vi "Measurement Logic.vi"() -> ()   [LabVIEW 2021, in "Single Tone_Audio DAC.lvlib"]
uses:
  Single Tone_Audio DAC.lvlib
  <vilib>/PDM Acquisition Toolkit/host/Classes/Channels/I2S Ouput/Controls/GenerationChannelProperties.ctl
  <vilib>/PDM Acquisition Toolkit/host/Classes/Channels/I2S Ouput/I2S Output Channel.lvclass
  <vilib>/PDM Acquisition Toolkit/host/Classes/Tasks/I2S Output/Control/SignalProperties.ctl
  <vilib>/PDM Acquisition Toolkit/host/Classes/Tasks/I2S Output/I2S Output Task.lvclass
  shared/controls/Digital Initialize Settings.ctl
  shared/controls/Analog Initialize Settings.ctl
  shared/controls/Single Tone Measurement Settings.ctl
  shared/controls/Single Tone Units.ctl
  Measurement Results.ctl
  shared/controls/Single Tone Filter Settings.ctl
  Measurement Configuration.ctl
  <vilib>/MeasurementLink/MeasurementLink Measurement Server/Measure Call Context/Measure Call Context.lvclass
panel:
  out "measure call context out":refnum<class "Measure Call Context.lvclass">
  in  "measure call context in":refnum<class "Measure Call Context.lvclass">
  out "measurement results":T1 {"Gain" format="%_6g"; "THD" format="%_6g"; "THD+N" format="%_6g"; "SNR" format="%_6g"; "SFDR (dBc)" format="%_6g"; "Dynamic range (dB)" format="%_6g"; "Phase (deg)" format="%_6g"; "Amplitude (dB)" format="%_6g"; "Amplitude (V)" format="%_6g"; "Frequency (Hz)" format="%_6g"; "df" format="%_6g"; "f0" format="%_6g"; "dt" format="%_6g"; "Frequency domain" format="%_6g"; "Time domain" format="%_6g"}
  in  "measurement configuration":T2={"Frequency (Hz)"=1000.0, "Protocol file"="C:\\Users\\Public\\Documents\\National Instruments\\AudioDAC\\ProtocolConfig\\I2SDEfault.dsgcfg", "Digital audio channel"="7821/PCMo 16", "Master clock channel"="7821/PCMo 24", "Output level"=0.0, "Output level units"="dBFS", "Output range (Vpk-pk)"=5.74, "Acquisition channel"="4468/ai0", "Sample rate (Hz)"=51200.0, "Min measurement cycles"=0, "Min measurement time (s)"=1.0, "Min settling cycles"=0, "Min settling time (s)"=0.5, "Highpass filter"="AC", "Lowpass filter"="AES17_20kHz", "Weighting filter"="A-weighting", "Band start (Hz)"=20.0, "Band stop (Hz)"=20000.0, "SNR units"="dB", "THD+N units"="dB", "THD units"="dB", "Gain units"="dB"} {"Band stop (Hz)" format="%#_6pHz"; "Band start (Hz)" format="%#_6pHz"; "Min settling time (s)" format="%#_6ps"; "Min measurement time (s)" format="%#_6ps"; "Sample rate (Hz)" format="%#_6pHz"; "Output range (Vpk-pk)" format="%.3p Vpk-pk"; "Output level" format="%#_6p"; "Frequency (Hz)" format="%#_6pHz"}
  out "error out":errorcluster
  in  "error in":errorcluster
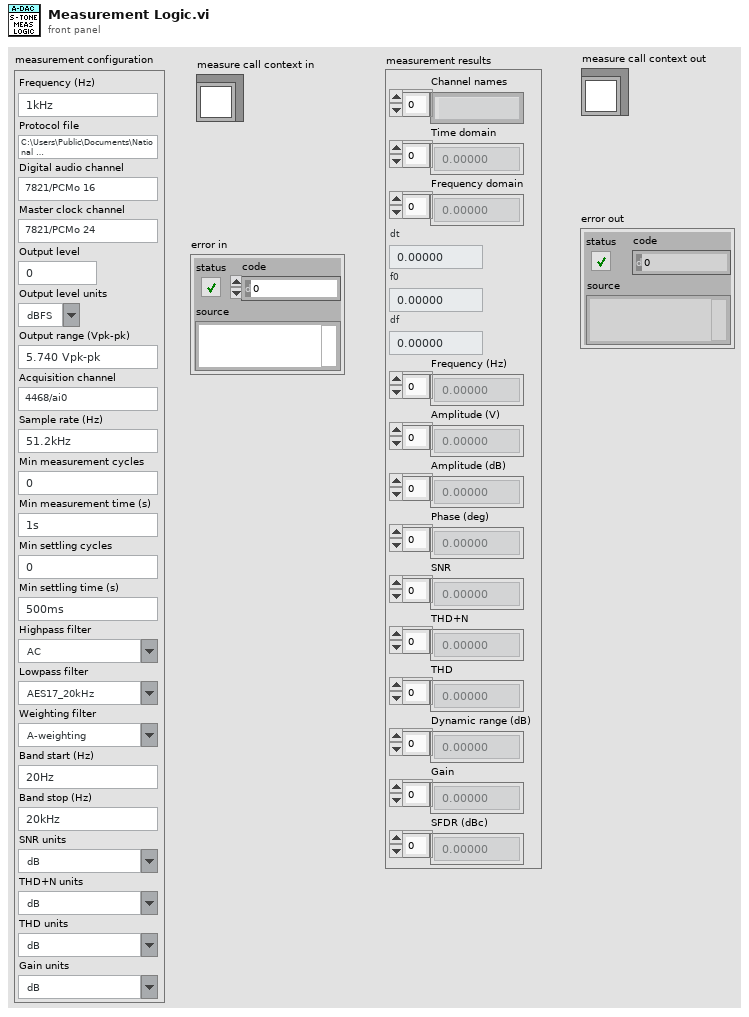
[diagram p1: front panel]
types:
  T1 = typedef "Single Tone_Audio DAC.lvlib/Measurement Results.ctl" = cluster{"Channel names":string[], "Time domain":dbl[], "Frequency domain":dbl[], "dt":dbl, "f0":dbl, "df":dbl, "Frequency (Hz)":dbl[], "Amplitude (V)":dbl[], "Amplitude (dB)":dbl[], "Phase (deg)":dbl[], "SNR":dbl[], "THD+N":dbl[], "THD":dbl[], "Dynamic range (dB)":dbl[], "Gain":dbl[], "SFDR (dBc)":dbl[]}
  T2 = typedef "Single Tone_Audio DAC.lvlib/Measurement Configuration.ctl" = cluster{"Frequency (Hz)":dbl, "Protocol file":string, "Digital audio channel":string, "Master clock channel":string, "Output level":dbl, "Output level units":string, "Output range (Vpk-pk)":dbl, "Acquisition channel":string, "Sample rate (Hz)":dbl, "Min measurement cycles":u32, "Min measurement time (s)":dbl, "Min settling cycles":u32, "Min settling time (s)":dbl, "Highpass filter":string, "Lowpass filter":string, "Weighting filter":string, "Band start (Hz)":dbl, "Band stop (Hz)":dbl, "SNR units":string, "THD+N units":string, "THD units":string, "Gain units":string}
  T3 = typedef "Single Tone Filter Settings.ctl" = cluster{"Highpass filter":string, "Lowpass filter":string, "Weighting filter":string}
  T4 = typedef "Single Tone Units.ctl" = cluster{"SNR units":string, "THD+N units":string, "THD units":string, "Gain units":string}
  T5 = typedef "Single Tone Measurement Settings.ctl" = cluster{"Band start":dbl, "Band stop":dbl, "Amplitude":dbl, "Frequency":dbl, "Full scale range":dbl}
  T6 = typedef "Analog Initialize Settings.ctl" = cluster{"analog acquisition channel":string, "samples per channel":i32, "sample rate":dbl}
  T7 = typedef "Digital Initialize Settings.ctl" = cluster{"digital channel list":string, "master clock channel list":string, "protocol settings file path":path, "signal parameters":T8}
  T8 = typedef "PDM Acquisition Class Library.lvlib/I2S Output Task.lvclass/SignalProperties.ctl" = cluster{"cyclic signal":dbl[], "channel parameters":T9[]}
  T9 = typedef "PDM Acquisition Class Library.lvlib/I2S Output Channel.lvclass/GenerationChannelProperties.ctl" = cluster{"cyclic period":dbl, "cyclic phase offset":dbl, "gain":dbl}
  T10 = typedef "PDM Acquisition Class Library.lvlib/PCM Output Task.lvclass/PCM Output Task DVR.ctl" = refnum<data-value>
  T11 = cluster{"channel":string, "frequency (Hz)":dbl, "amplitude (Vrms)":dbl, "amplitude (dBFS)":dbl, "phase (deg)":dbl, "SNR":dbl, "THD+N":dbl, "THD":dbl, "dynamic range (dB)":dbl, "gain":dbl, "SFDR (dBc)":dbl}[]
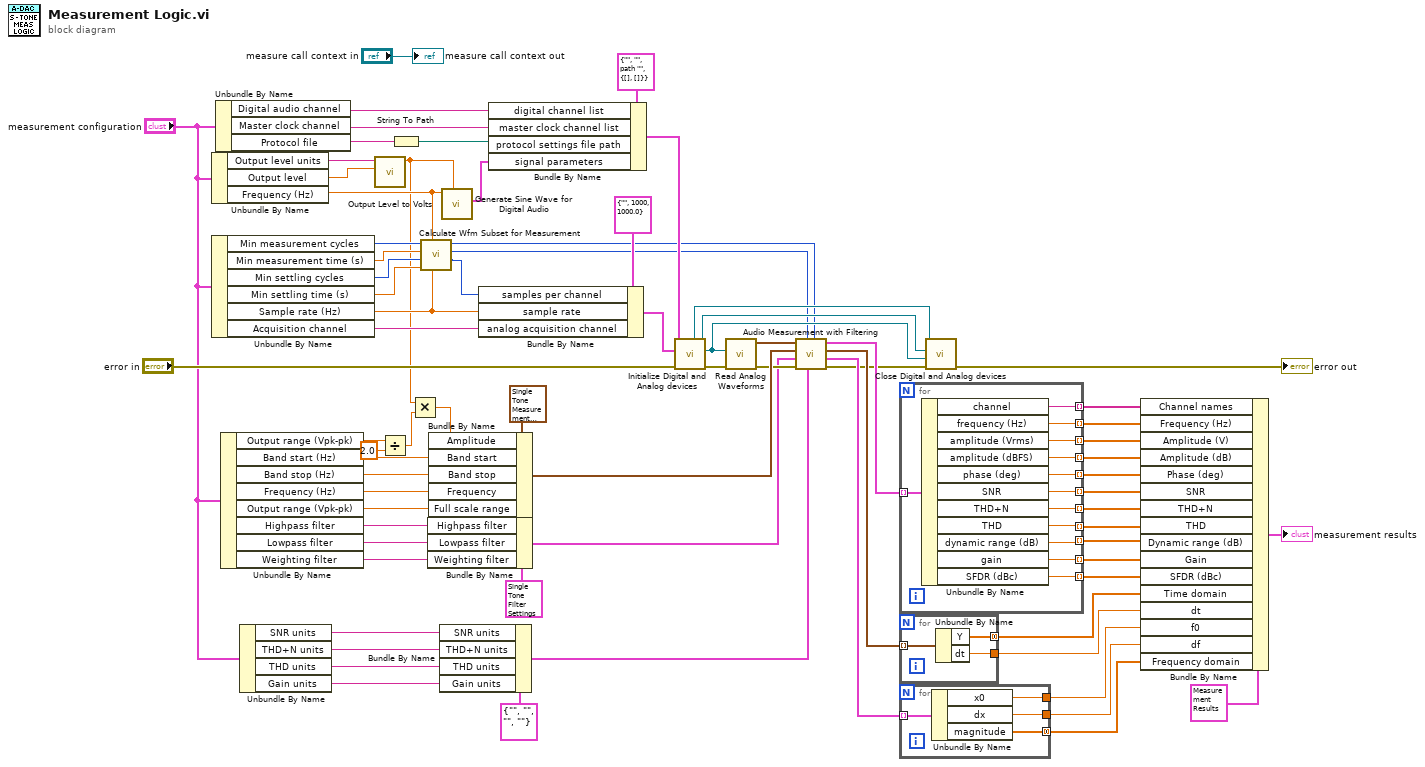
[diagram p0: block diagram]
diagram:
  n1 = Unbundle By Name("measurement configuration") -> ("Output level units"=w74:string, "Output level"=w73:dbl, "Frequency (Hz)"=w45:dbl)
  n2 = Unbundle By Name("measurement configuration") -> ("Min measurement cycles"=w72:u32, "Min measurement time (s)"=w71:dbl, "Min settling cycles"=w70:u32, "Min settling time (s)"=w69:dbl, "Sample rate (Hz)"=w58:dbl, "Acquisition channel"=w59:string)
  n3 = Unbundle By Name("measurement configuration") -> ("Digital audio channel"=w67:string, "Master clock channel"=w66:string, "Protocol file"=w65:string)
  n4 = Unbundle By Name("measurement configuration") -> ("Output range (Vpk-pk)"=w26:dbl, "Band start (Hz)"=w54:dbl, "Band stop (Hz)"=w53:dbl, "Frequency (Hz)"=w52:dbl, "Output range (Vpk-pk)"=w51:dbl, "Highpass filter"=w7:string, "Lowpass filter"=w6:string, "Weighting filter"=w5:string)
  n5 = Unbundle By Name("measurement configuration") -> ("SNR units"=w12:string, "THD+N units"=w11:string, "THD units"=w10:string, "Gain units"=w9:string)
  n6 = call "Output Level to Volts.vi"("Output level in"=w73, "Output level units"=w74) -> ("Output level out"=w23:dbl)  [unwired: 9 in]
  n7 = Divide(x=w26, y=2.0) -> (x/y=w24:dbl)
  n8 = String To Path(string=w65) -> (path=w64:path)
  n9 = Multiply(x=w23, y=w24) -> (x*y=w22:dbl)
  n10 = call "Calculate Wfm Subset for Measurement.vi"("sampling rate"=w58, "signal frequency"=w45, "minimum settling duration"=w69, "minimum settling cycles"=w70, "minimum measurement duration"=w71, "minimum measurement cycles"=w72) -> ("total acquisition (samples)"=w3:u32, "duration (samples)"=w1:u32, "start (samples)"=w2:u32)  [unwired: 3 in]
  n11 = Bundle By Name(cluster=T3 {"Highpass filter"="DC", "Lowpass filter"="No filter", "Weighting filter"="A-weighting"} ("filter settings"), "Highpass filter"=w7, "Lowpass filter"=w6, "Weighting filter"=w5) -> (w4:T3)
  n12 = Bundle By Name(cluster=T5 {"Band start"=20.0, "Band stop"=20000.0, "Amplitude"=1.0, "Frequency"=1000.0, "Full scale range"=3.16} ("measurement settings"), "Amplitude"=w22, "Band start"=w54, "Band stop"=w53, "Frequency"=w52, "Full scale range"=w51) -> (w20:T5)
  n13 = Bundle By Name(cluster=T4 {"SNR units"="", "THD+N units"="", "THD units"="", "Gain units"=""} ("units"), "SNR units"=w12, "THD+N units"=w11, "THD units"=w10, "Gain units"=w9) -> (w19:T4)
  n14 = call "Generate Sine Wave for Digital Audio.vi"("gain"=w23, "frequency"=w45) -> ("Signal Properties"=w63:T8)  [unwired: 9 in]
  n15 = Bundle By Name(cluster=T6 {"analog acquisition channel"="", "samples per channel"=1000, "sample rate"=1000.0} ("Analog initialize settings"), "samples per channel"=w3, "sample rate"=w58, "analog acquisition channel"=w59) -> (w57:T6)
  n16 = Bundle By Name(cluster=T7 {"digital channel list"="", "master clock channel list"="", "protocol settings file path"=path "", "signal parameters"={"cyclic signal"=[], "channel parameters"=[]}} ("Digital initialize settings"), "digital channel list"=w67, "master clock channel list"=w66, "protocol settings file path"=w64, "signal parameters"=w63) -> (w61:T7)
  n17 = call "Initialize Digital and Analog devices.vi"("error in"="error in", "Analog initialize settings"=w57, "Digital initialize settings"=w61) -> ("error out"=w56:errorcluster, "analog task"=w47:refnum<k21>, "master clock task"=w49:T10, "digital audio task"=w48:T10)  [unwired: 5 in]
  n18 = call "Read Analog Waveforms.vi"("error in"=w56, "analog task"=w47) -> ("error out"=w14:errorcluster, "waveforms"=w21:waveform(dbl)[])  [unwired: 7 in, 1 out]
  n19 = call "Audio Measurement with Filtering.vi"("start"=w2, "units"=w19, "duration"=w1, "error in"=w14, "filter settings"=w4, "measurement settings"=w20, "waveforms"=w21) -> ("error out"=w15:errorcluster, "spectra"=w16:cluster{"x0":dbl, "dx":dbl, "magnitude":dbl[]}[], "time domain"=w17:waveform(dbl)[], "results"=w18:T11)  [unwired: 1 in]
  n20 = for {
    tunnel: w18 -> [w87] mode=indexing
    tunnel: [w86] -> w43 mode=indexing
    tunnel: [w85] -> w42 mode=indexing
    tunnel: [w84] -> w41 mode=indexing
    tunnel: [w83] -> w40 mode=indexing
    tunnel: [w82] -> w39 mode=indexing
    tunnel: [w81] -> w38 mode=indexing
    tunnel: [w80] -> w37 mode=indexing
    tunnel: [w79] -> w36 mode=indexing
    tunnel: [w78] -> w35 mode=indexing
    tunnel: [w77] -> w34 mode=indexing
    tunnel: [w76] -> w33 mode=indexing
    n21 = Unbundle By Name(w87) -> ("channel"=w86:string, "frequency (Hz)"=w85:dbl, "amplitude (Vrms)"=w84:dbl, "amplitude (dBFS)"=w83:dbl, "phase (deg)"=w82:dbl, "SNR"=w81:dbl, "THD+N"=w80:dbl, "THD"=w79:dbl, "dynamic range (dB)"=w78:dbl, "gain"=w77:dbl, "SFDR (dBc)"=w76:dbl)
  }
  n22 = for {
    tunnel: w17 -> [w90] mode=indexing
    tunnel: [w89] -> w32 mode=concatenating
    tunnel: [w88] -> w31
    n23 = Unbundle By Name(w90) -> ("Y"=w89:dbl[], "dt"=w88:dbl)
  }
  n24 = for {
    tunnel: w16 -> [w94] mode=indexing
    tunnel: [w93] -> w30
    tunnel: [w92] -> w29
    tunnel: [w91] -> w28 mode=concatenating
    n25 = Unbundle By Name(w94) -> ("x0"=w93:dbl, "dx"=w92:dbl, "magnitude"=w91:dbl[])
  }
  n26 = call "Close Digital and Analog devices.vi"("error in"=w15, "analog task"=w47, "master clock task"=w49, "digital audio task"=w48) -> ("error out"=→"error out":errorcluster)  [unwired: 7 in]
  n27 = Bundle By Name(cluster=T1 {"Channel names"=[], "Time domain"=[], "Frequency domain"=[], "dt"=0.0, "f0"=0.0, "df"=0.0, "Frequency (Hz)"=[], "Amplitude (V)"=[], "Amplitude (dB)"=[], "Phase (deg)"=[], "SNR"=[], "THD+N"=[], "THD"=[], "Dynamic range (dB)"=[], "Gain"=[], "SFDR (dBc)"=[]} ("measurement results"), "Channel names"=w43, "Frequency (Hz)"=w42, "Amplitude (V)"=w41, "Amplitude (dB)"=w40, "Phase (deg)"=w39, "SNR"=w38, "THD+N"=w37, "THD"=w36, "Dynamic range (dB)"=w35, "Gain"=w34, "SFDR (dBc)"=w33, "Time domain"=w32, "dt"=w31, "f0"=w30, "df"=w29, "Frequency domain"=w28) -> (→"measurement results":T1)
  "measure call context out" <- "measure call context in"
